vi "Run Command.vi"(2 "Line Index In":i32, 3 "Script":string) -> (0 "Line Index Out":i32, 1 "Done":bool)   [LabVIEW 2013]
doc: "Looks at a line and runs the appropriate command. Add new commands to this vi."
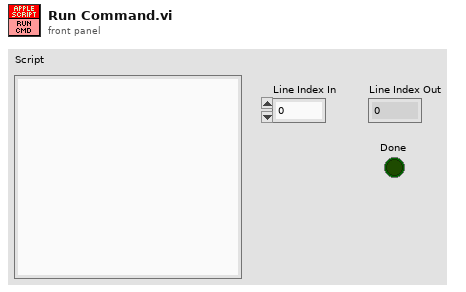
[diagram p1: front panel]
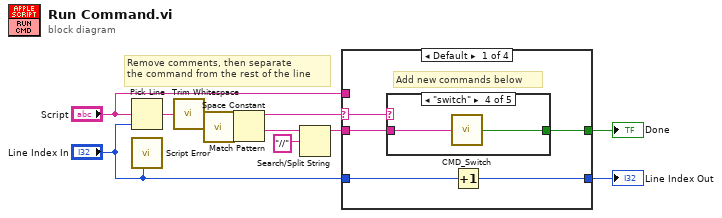
[diagram p0: block diagram]
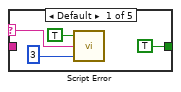
[diagram p2: hidden frame]
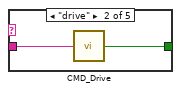
[diagram p3: hidden frame]
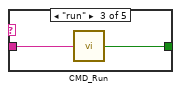
[diagram p4: hidden frame]
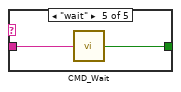
[diagram p5: hidden frame]
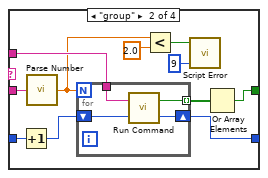
[diagram p6: hidden frame]
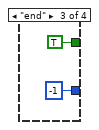
[diagram p7: hidden frame]
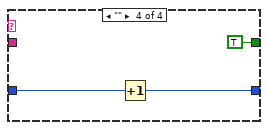
[diagram p8: hidden frame]
diagram:
  # "Remove comments, then separate\nthe command from the rest of the line"
  n1 = Pick Line(multi-line string="Script", line index="Line Index In") -> (output string=w4:string)  [unwired: 1 in]
  n2 = call "Script Error.vi"("Line Number"="Line Index In") -> ()  [unwired: 5 in]
  n3 = call <vilib>:"Trim Whitespace.vi"("string"=w4) -> ("trimmed string"=w3:string)  [unwired: 1 in]
  n4 = call <vilib>:"Space Constant.vi"() -> ("String"=w11:string)
  n5 = Match Pattern(string=w3, regular expression=w11) -> (before substring=w10:string, after substring=w5:string)  [unwired: 1 in, 2 out]
  n6 = Search/Split String(string=w5, search string/char (-)="//") -> (substring before match=w2:string)  [unwired: 1 in, 2 out]
  n7 = case shown="Default" w10 {
    selector: w10 -> [w14 _ _ _]
    tunnel: "Script" -> [_ w38 _ _]
    tunnel: "Line Index In" -> [w16 w34 _ w47]
    tunnel: [w13 w36 TRUE ("Running") TRUE ("Running")] -> w8
    tunnel: [w15 w35 -1 ("Line Index Out") w46] -> w7
    tunnel: w2 -> [w12 w39 _ _]
    frame Default {
      # "Add new commands below"
      n8 = case shown="\"switch\"" w14 {
        selector: w14 -> [w17 _ _ _ _]
        tunnel: [TRUE w22 w24 w25 w27] -> w13
        tunnel: w12 -> [_ w21 w23 w26 w28]
        frame Default {
          n9 = call "Script Error.vi"("Error?"=TRUE, "Error Details"=w17, "Error Code"=3) -> ()  [unwired: 3 in]
        }
        frame "drive" {
          n10 = call "CMD_Drive.vi"("Line"=w21) -> ("Done"=w22:bool)
        }
        frame "run" {
          n11 = call "CMD_Run.vi"("Line"=w23) -> ("Done"=w24:bool)
        }
        frame "switch" {
          n12 = call "CMD_Switch.vi"("Line"=w26) -> ("Done"=w25:bool)
        }
        frame "wait" {
          n13 = call "CMD_Wait.vi"("Line"=w28) -> ("Done"=w27:bool)
        }
      }
      n14 = Increment(x=w16) -> (x+1=w15:i32)
    }
    frame "group" {
      n15 = Increment(x=w34) -> (x+1=w33:i32)
      n16 = call "Parse Number.vi"("String"=w39) -> ("Number"=w31:dbl)
      n17 = for {
        N: w31 -> [_]
        tunnel: w38 -> [w43]
        tunnel: [w42] -> w37 mode=indexing
        shift-right: [w41] -> w35
        shift-left: w33 -> [w40]
        n18 = call "Run Command.vi"("Line Index In"=w40, "Script"=w43) -> ("Line Index Out"=w41:i32, "Done"=w42:bool)
      }
      n19 = Less?(x=w31, y=2.0) -> (x < y?=w30:bool)
      n20 = call "Script Error.vi"("Error?"=w30, "Error Code"=9) -> ()  [unwired: 4 in]
      n21 = Or Array Elements(Boolean array=w37) -> (logical OR=w36:bool)
    }
    frame "end" {
    }
    frame "" {
      n22 = Increment(x=w47) -> (x+1=w46:i32)
    }
  }
  "Line Index Out" <- w7
  "Done" <- w8
